vi "Search.vi"(6 "Index in":i32=-1, 7 "Composite Object":refnum<class "CConfig Object.lvclass">, 8 "error in (no error)":errorcluster, 11 "Find Query in":refnum<class "All Query.lvclass">) -> (0 "error out":errorcluster, 2 "empty?":bool, 3 "Find Query out":refnum<class "All Query.lvclass">, 5 "Composite Object":refnum<class "CConfig Object.lvclass">)   [LabVIEW 2013, in "All Query.lvclass"]
doc: "Copyright 2018, Carya Automatisering, Wiebe Walstra."
uses:
  All Query.lvclass
  CConfig Object.lvclass
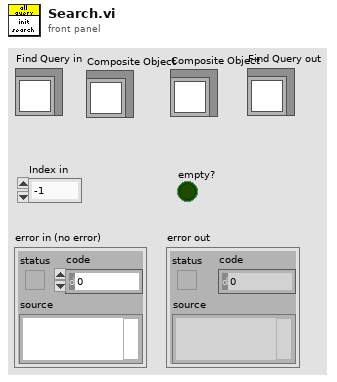
[diagram p1: front panel]
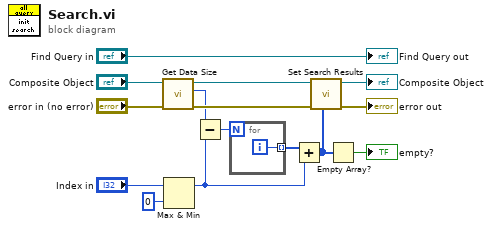
[diagram p0: block diagram]
diagram:
  n1 = call-dynamic "Get Data Size.vi"("error in (no error)"="error in (no error)", "Composite Object in"="Composite Object") -> ("error out"=w7:errorcluster, "Elements"=w3:i32, "Composite Object out"=w6:refnum<class "CConfig Object.lvclass">)  [unwired: 7 in]
  n2 = Max & Min(x="Index in", y=0) -> (max(x,y)=w2:i32)  [unwired: 1 out]
  n3 = Subtract(x=w3, y=w2) -> (x-y=w1:i32)
  n4 = for {
    N: w1 -> [_]
    tunnel: [w16] -> w10 mode=indexing
    i -> [w16]
  }
  n5 = Add(x=w10, y=w2) -> (x+y=w8:i32[])
  n6 = call-dynamic "Set Search Results.vi"("Search results"=w8, "error in (no error)"=w7, "Composite Object in"=w6) -> ("error out"=→"error out":errorcluster, "Composite Object out"=→"Composite Object":refnum<class "CConfig Object.lvclass">)  [unwired: 7 in]
  n7 = Empty Array?(array=w8) -> (empty?=→"empty?":bool)
  "Find Query out" <- "Find Query in"
